vi "Recieve MSG.vi"(2 "Stop":bool, 3 "N":u8=1, 4 "error in":errorcluster {"code" format="%.0x"}, 5 "CAN Channal Handle":u32) -> (0 "CAN Channel Handle out":u32, 1 "MSG  array":T1(array[cluster]))   [LabVIEW 2011]
panel:
  out "PrevID":u16[](array[numeric])
  out "K":u32
  out "Data Start":bool=TRUE
  out "error out":errorcluster {"code" format="%.0x"}
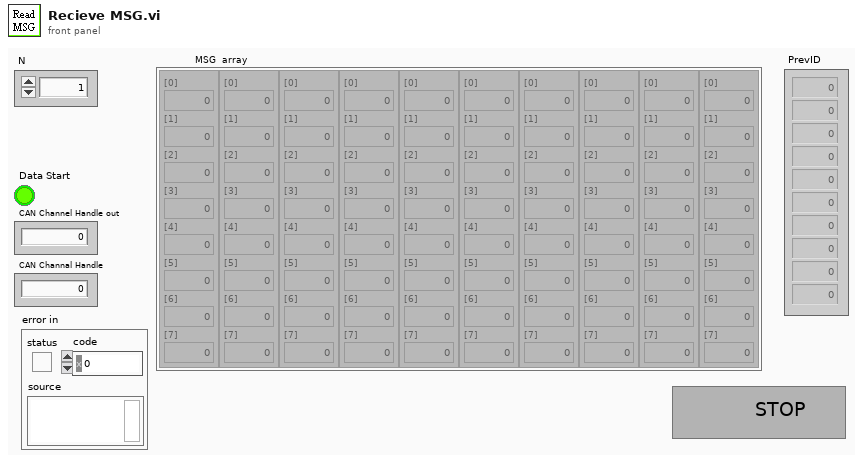
[diagram p1: front panel]
types:
  T1 = cluster{"[0]":u8, "[1]":u8, "[2]":u8, "[3]":u8, "[4]":u8, "[5]":u8, "[6]":u8, "[7]":u8}[]
  T2 = cluster{"[0]":u8, "[1]":u8, "[2]":u8, "[3]":u8, "[4]":u8, "[5]":u8, "[6]":u8, "[7]":u8}
  T3 = cluster{"Timestamp":u32, "Arbitration ID":u32, "DLC":u8, "Type":enum8{"data", "info", "error", "status", "wakeup", "timer ovr", "timer reset"}, "AFC":enum8{"reject", "always", "filter 1", "filter 2"}, "extended frame":bool, "remote request":bool, "self reception":bool, "receive buffer full":bool, "Data":cluster{"[0]":u8, "[1]":u8, "[2]":u8, "[3]":u8, "[4]":u8, "[5]":u8, "[6]":u8, "[7]":u8}}
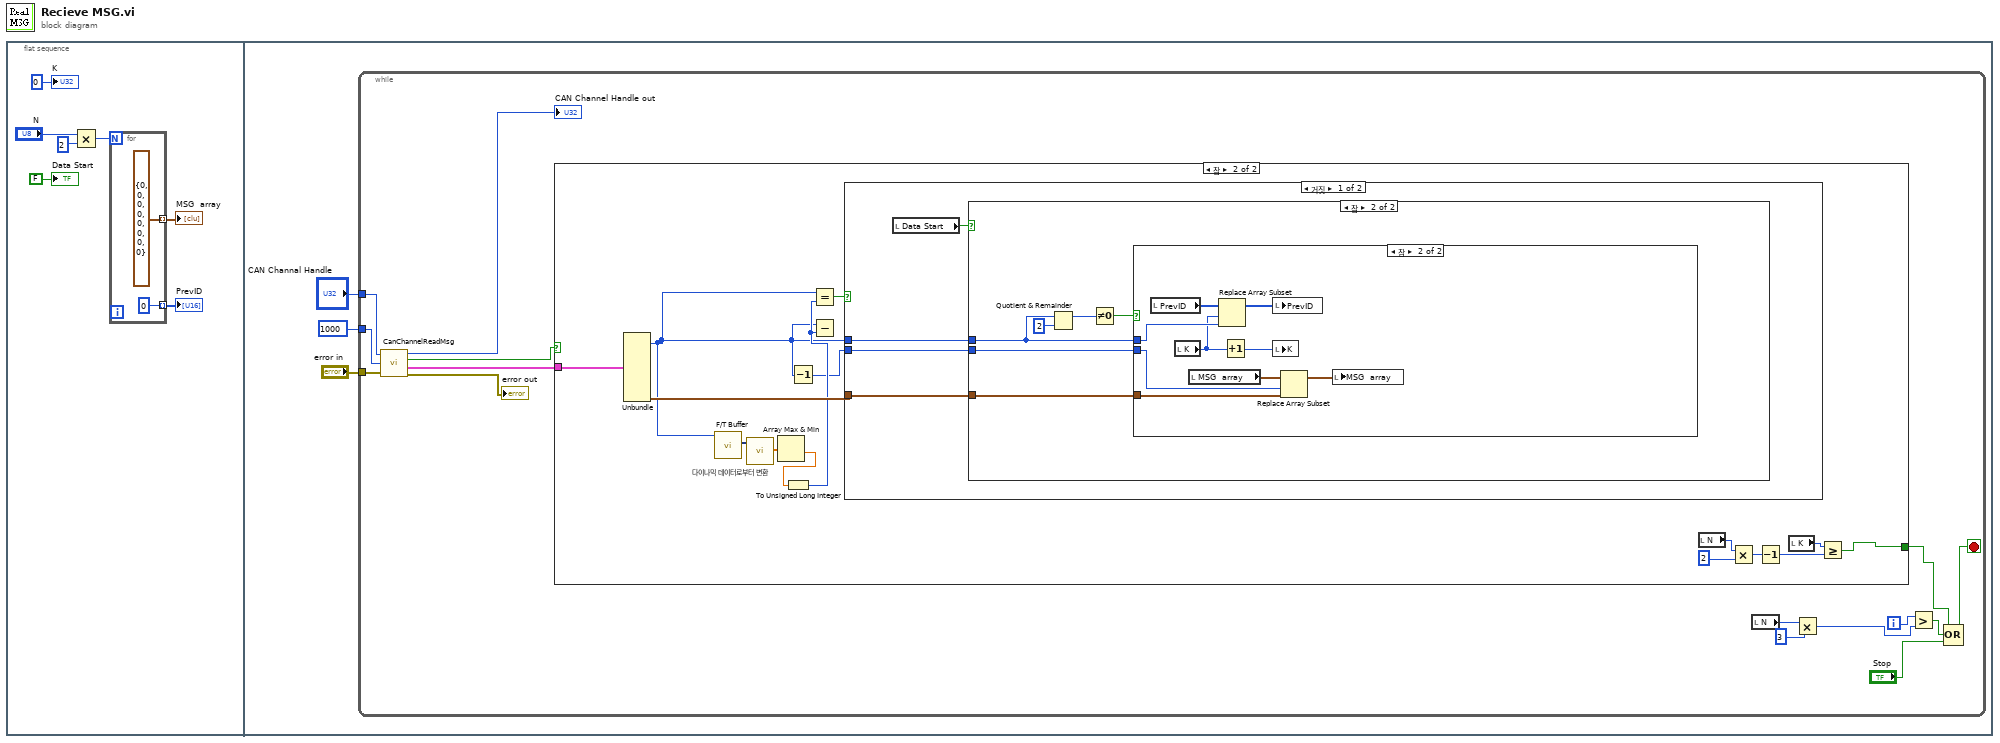
[diagram p0: block diagram]
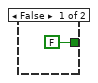
[diagram p2: hidden frame]
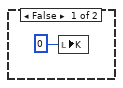
[diagram p3: hidden frame]
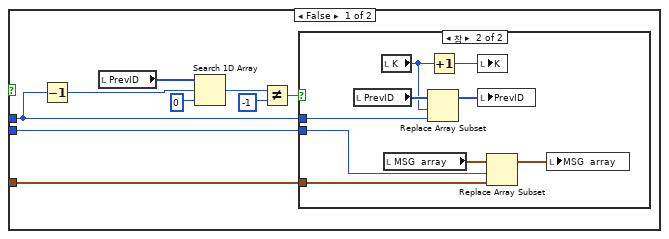
[diagram p4: hidden frame]
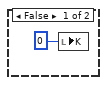
[diagram p5: hidden frame]
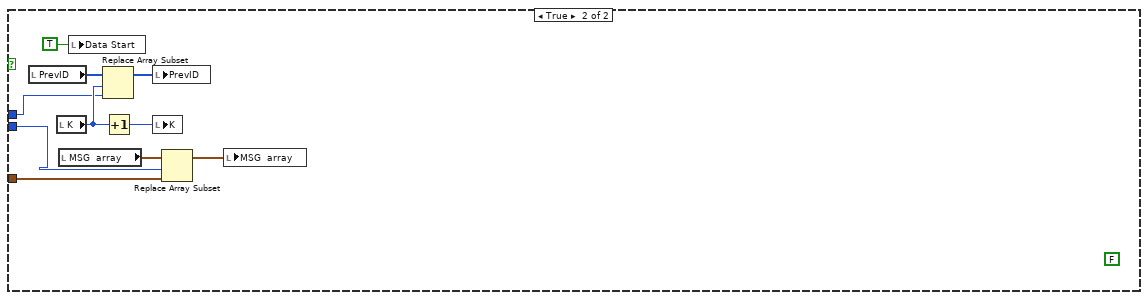
[diagram p6: hidden frame]
diagram:
  n1 = flat-sequence {
    frame #0 {
      n2 = Multiply(x="N", y=u8 2) -> (x*y=w5:u8)
      n3 = for {
        N: w5 -> [_]
        tunnel: [T2 {"[0]"=0, "[1]"=0, "[2]"=0, "[3]"=0, "[4]"=0, "[5]"=0, "[6]"=0, "[7]"=0} ("Data")] -> w4 mode=indexing
        tunnel: [u16 0 ("Numeric")] -> w1 mode=indexing
      }
      "MSG  array" <- w4
      "PrevID" <- w1
      "Data Start" <- FALSE ("불리언 3")
      "K" <- u32 0 ("K")
    }
    frame #1 {
      n4 = while {
        tunnel: "error in" -> [w26]
        tunnel: "CAN Channal Handle" -> [w25]
        tunnel: u32 1000 ("Milliseconds") -> [w24]
        i -> [w20]
        stop <- w13 stop-if-true
        n5 = call "CanChannelReadMsg.vi"("CAN Channel Handle in"=w25, "Milliseconds"=w24, "error in"=w26) -> ("CAN Channel Handle out"=→"CAN Channel Handle out":u32, "Is Valid Message"=w22:bool, "CAN message"=w21:T3, "error out"=→"error out":errorcluster)
        n6 = case shown="참" w22 {
          tunnel: w21 -> [_ w43]
          tunnel: [FALSE ("불리언 3") w29] -> w16
          frame False {
          }
          frame True {
            n7 = Unbundle(w43) -> ("Arbitration ID"=w31:u32, "Data"=w42:T2)  [unwired: 8 out]
            n8 = call "F/T Buffer"("Signals"=w31) -> ("Collected Signals"=w35:dynamicdata)  [unwired: 9 in, 1 out]
            n9 = call "다이나믹 데이터로부터 변환"("Dynamic Data Type"=w35) -> ("Array"=w34:dbl[])  [unwired: 3 in]
            n10 = Array Max & Min(array=w34) -> (min value=w33:dbl)  [unwired: 3 out]
            n11 = To Unsigned Long Integer(number=w33) -> (unsigned 32bit integer=w32:u32)
            n12 = Decrement(x=w31) -> (x-1=w30:u32)
            n13 = Equal?(x=w31, y=w32) -> (x = y?=w41:bool)
            n14 = Subtract(x=w31, y=w32) -> ()  [unwired: 1 out]
            n15 = case shown="거짓" w41 {
              tunnel: w31 -> [w47 w87]
              tunnel: w42 -> [w46 w86]
              tunnel: w30 -> [w44 w83]
              frame False {
                n16 = local read "Data Start"() -> (w45:bool)
                n17 = case shown="참" w45 {
                  tunnel: w47 -> [_ w51]
                  tunnel: w46 -> [_ w50]
                  tunnel: w44 -> [_ w49]
                  frame False {
                    n18 = local write "K"(u32 0 ("K")) -> ()
                  }
                  frame True {
                    n19 = Quotient & Remainder(x=w51, y=u32 2) -> (x-y*floor(x/y)=w53:u32)  [unwired: 1 out]
                    n20 = Not Equal To 0?(x=w53) -> (x != 0?=w52:bool)
                    n21 = case shown="참" w52 {
                      tunnel: w51 -> [w57 w76]
                      tunnel: w50 -> [w56 w80]
                      tunnel: w49 -> [w55 w74]
                      frame False {
                        n22 = Decrement(x=w57) -> (x-1=w63:u32)
                        n23 = local read "PrevID"() -> (w62:u16[])
                        n24 = Search 1D Array(1D array=w62, element=w63, start index (0)=0 ("시작 인덱스(0)")) -> (index of element=w60:i32)
                        n25 = Not Equal?(x=w60, y=-1) -> (x != y?=w58:bool)
                        n26 = case shown="참" w58 {
                          tunnel: w57 -> [_ w67]
                          tunnel: w56 -> [_ w66]
                          tunnel: w55 -> [_ w65]
                          frame False {
                            n27 = local write "K"(u32 0 ("K")) -> ()
                          }
                          frame True {
                            n28 = local read "PrevID"() -> (w73:u16[])
                            n29 = local read "K"() -> (w70:u32)
                            n30 = local read "MSG  array"() -> (w69:T1)
                            n31 = Replace Array Subset(array=w73, new element=w67, index=w70) -> (w72:u16[])
                            n32 = Increment(x=w70) -> (x+1=w71:u32)
                            n33 = local write "K"(w71) -> ()
                            n34 = local write "PrevID"(w72) -> ()
                            n35 = Replace Array Subset(array=w69, new element=w66, index=w65) -> (w68:T1)
                            n36 = local write "MSG  array"(w68) -> ()
                          }
                        }
                      }
                      frame True {
                        n37 = local read "PrevID"() -> (w78:u16[])
                        n38 = local read "K"() -> (w75:u32)
                        n39 = local read "MSG  array"() -> (w82:T1)
                        n40 = Replace Array Subset(array=w78, new element=w76, index=w75) -> (w77:u16[])
                        n41 = Increment(x=w75) -> (x+1=w79:u32)
                        n42 = local write "PrevID"(w77) -> ()
                        n43 = local write "K"(w79) -> ()
                        n44 = Replace Array Subset(array=w82, new element=w80, index=w74) -> (w81:T1)
                        n45 = local write "MSG  array"(w81) -> ()
                      }
                    }
                  }
                }
              }
              frame True {
                (unwired) FALSE ("Data Start")
                n46 = local read "PrevID"() -> (w91:u16[])
                n47 = local read "K"() -> (w90:u32)
                n48 = local read "MSG  array"() -> (w88:T1)
                n49 = local write "Data Start"(TRUE ("Data Start")) -> ()
                n50 = Replace Array Subset(array=w91, new element=w87, index=w90) -> (w89:u16[])
                n51 = Increment(x=w90) -> (x+1=w92:u32)
                n52 = local write "PrevID"(w89) -> ()
                n53 = local write "K"(w92) -> ()
                n54 = Replace Array Subset(array=w88, new element=w86, index=w83) -> (w85:T1)
                n55 = local write "MSG  array"(w85) -> ()
              }
            }
            n56 = local read "N"() -> (w40:u8)
            n57 = Multiply(x=w40, y=u32 2) -> (x*y=w38:u32)
            n58 = Decrement(x=w38) -> (x-1=w37:u32)
            n59 = local read "K"() -> (w36:u32)
            n60 = Greater Or Equal?(x=w36, y=w37) -> (x >= y?=w29:bool)
          }
        }
        n61 = local read "N"() -> (w19:u8)
        n62 = Multiply(x=w19, y=u8 3) -> (x*y=w17:u8)
        n63 = Greater?(x=w20, y=w17) -> (0:w15:bool)
        n64 = Compound Arithmetic op=OR(w16, w15, "Stop") -> (w13:bool)
      }
    }
  }
